vi "Calculator Brainstorming V4.vi"() -> ()   [LabVIEW 2017]
doc: "This is a calculator designed for physics students. It features 7 commonly used physics constants, and the 4 usual operators."
panel:
  in  "=":bool
  in  "÷":bool
  in  "x":bool
  in  "-":bool
  in  "+":bool
  in  "0 8":bool
  in  "Pi":bool
  in  "0 7":bool
  in  "mp":bool
  in  "me":bool
  in  "G":bool
  in  "C":bool
  in  ".":bool
  in  "9":bool
  in  "8":bool
  in  "7":bool
  in  "0":bool
  in  "6":bool
  in  "?":bool
  in  "?":bool
  in  "1":bool
  in  "5":bool
  in  "4":bool
  in  "3":bool
  in  "2":bool
  out "Display":dbl
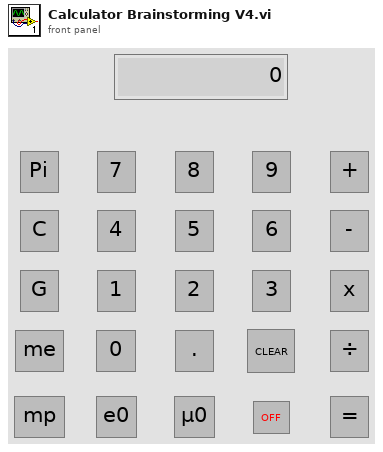
[diagram p1: front panel]
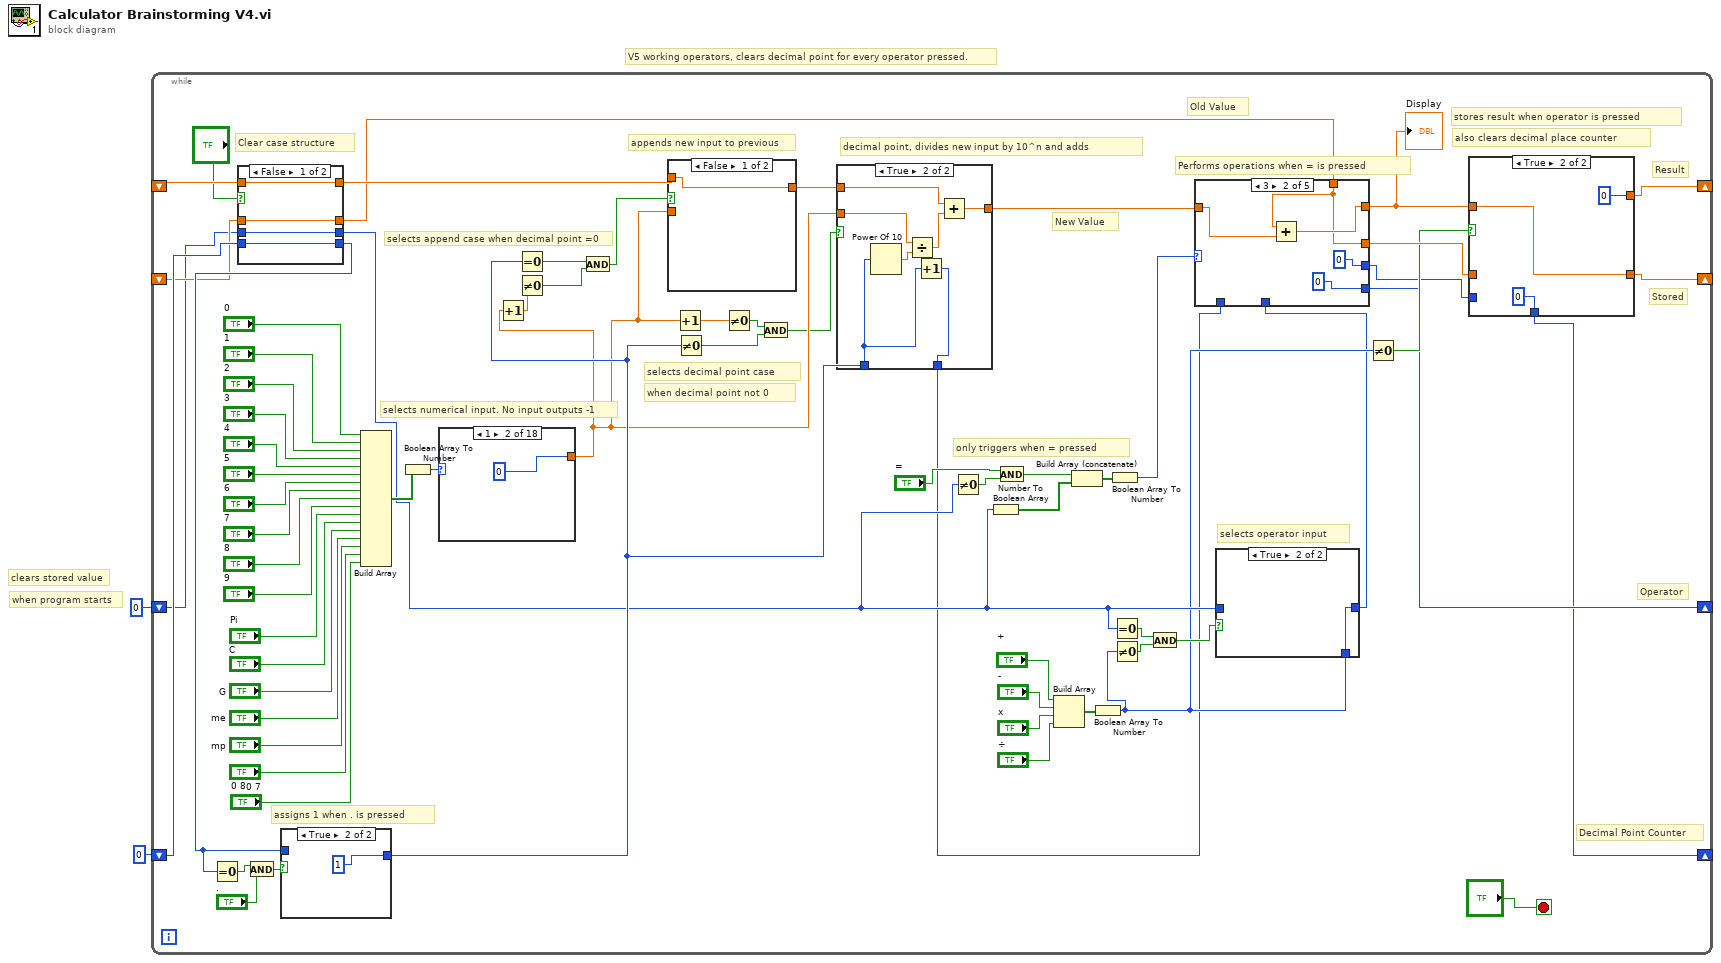
[diagram p0: block diagram]
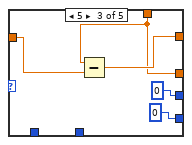
[diagram p4: hidden frame]
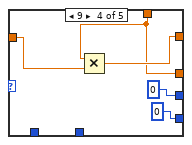
[diagram p5: hidden frame]
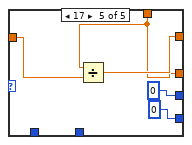
[diagram p6: hidden frame]
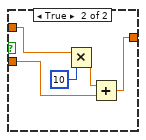
[diagram p8: hidden frame]
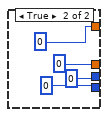
[diagram p11: hidden frame]
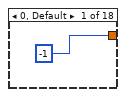
[diagram p12: hidden frame]
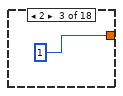
[diagram p13: hidden frame]
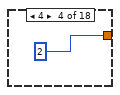
[diagram p14: hidden frame]
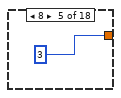
[diagram p15: hidden frame]
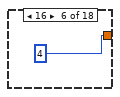
[diagram p16: hidden frame]
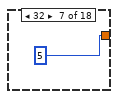
[diagram p17: hidden frame]
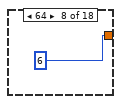
[diagram p18: hidden frame]
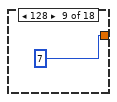
[diagram p19: hidden frame]
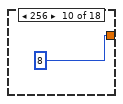
[diagram p20: hidden frame]
diagram:
  # "when program starts"
  # "clears stored value"
  # "V5 working operators, clears decimal point for every operator pressed."
  n1 = while {
    shift-right: [w16] -> _
    shift-left: _ -> [w69]
    shift-right: [w4] -> _
    shift-left: 0 -> [w52]
    shift-right: [w17] -> _
    shift-left: _ -> [w34]
    shift-right: [w7] -> _
    shift-left: 0 -> [w32]
    stop <- "?" stop-if-true
    # "Clear case structure"
    # "when decimal point not 0"
    # "selects decimal point case"
    # "selects append case when decimal point =0"
    # "also clears decimal place counter"
    # "stores result when operator is pressed"
    # "Performs operations when = is pressed"
    # "assigns 1 when . is pressed"
    # "only triggers when = pressed"
    # "selects operator input"
    # "decimal point, divides new input by 10^n and adds"
    # "New Value"
    # "Old Value"
    # "Operator"
    # "Stored"
    # "Decimal Point Counter"
    # "appends new input to previous"
    # "selects numerical input. No input outputs -1"
    # "Result"
    n2 = case shown="False" "?" {
      tunnel: [w124 0] -> w33
      tunnel: w69 -> [w124 _]
      tunnel: [w123 0] -> w53
      tunnel: w52 -> [w123 _]
      tunnel: [w122 0] -> w27
      tunnel: w34 -> [w122 _]
      tunnel: [w121 0] -> w12
      tunnel: w32 -> [w121 _]
      frame False {
      }
      frame True {
      }
    }
    n3 = Equal To 0?(x=w53) -> (x = 0?=w55:bool)
    n4 = And(x=w55, y=".") -> (x .and. y?=w56:bool)
    n5 = case shown="True" w56 {
      tunnel: w53 -> [w119 _]
      tunnel: [w119 1] -> w47
      frame False {
      }
      frame True {
      }
    }
    n6 = Build Array("0", "1", "2", "3", "4", "5", "6", "7", "8", "9", "Pi", "C", "G", "me", "mp", "0 7", "0 8") -> (w67:bool[])
    n7 = Boolean Array To Number(Boolean array=w67) -> (number=w71:u32)
    n8 = case shown="1" w71 {
      tunnel: [-1 0 1 2 3 4 5 6 7 8 9 3.141592653589793 w142 w144 9.10938356e-31 1.6726219e-27 8.85418782e-12 1.25663706e-06] -> w46
      frame 0, Default {
      }
      frame 1 {
      }
      frame 2 {
      }
      frame 4 {
      }
      frame 8 {
      }
      frame 16 {
      }
      frame 32 {
      }
      frame 64 {
      }
      frame 128 {
      }
      frame 256 {
      }
      frame 512 {
      }
      frame 1024 {
      }
      frame 2048 {
        # "cast to remove units"
        n9 = Cast Unit Bases(0:ext[unit] 299792458.0) -> (2:w142:ext)  [unwired: 1 in]
      }
      frame 4096 {
        n10 = Cast Unit Bases(0:ext[unit] 6.67408e-11) -> (2:w144:ext)  [unwired: 1 in]
      }
      frame 8192 {
      }
      frame 16384 {
      }
      frame 32768 {
      }
      frame 65536 {
      }
    }
    n11 = Increment(x=w46) -> (x+1=w49:ext)
    n12 = Equal To 0?(x=w47) -> (x = 0?=w48:bool)
    n13 = Not Equal To 0?(x=w49) -> (x != 0?=w50:bool)
    n14 = And(x=w48, y=w50) -> (x .and. y?=w3:bool)
    n15 = case shown="False" w3 {
      tunnel: w33 -> [w104 w107]
      tunnel: [w104 w106] -> w51
      tunnel: w46 -> [_ w105]
      frame False {
      }
      frame True {
        n16 = Multiply(x=w107, y=10) -> (x*y=w109:ext)
        n17 = Add(x=w109, y=w105) -> (x+y=w106:ext)
      }
    }
    n18 = Increment(x=w46) -> (x+1=w42:ext)
    n19 = Not Equal To 0?(x=w47) -> (x != 0?=w44:bool)
    n20 = Not Equal To 0?(x=w42) -> (x != 0?=w45:bool)
    n21 = And(x=w45, y=w44) -> (x .and. y?=w43:bool)
    n22 = case shown="True" w43 {
      tunnel: w51 -> [w111 w116]
      tunnel: [w111 w115] -> w23
      tunnel: w47 -> [w110 w113]
      tunnel: w46 -> [_ w114]
      tunnel: [w110 w112] -> w6
      frame False {
      }
      frame True {
        n23 = Power Of 10(x=w113) -> (10^x=w118:dbl)
        n24 = Divide(x=w114, y=w118) -> (x/y=w117:ext)
        n25 = Increment(x=w113) -> (x+1=w112:i32)
        n26 = Add(x=w116, y=w117) -> (x+y=w115:ext)
      }
    }
    n27 = Not Equal To 0?(x=w12) -> (x != 0?=w25:bool)
    n28 = Number To Boolean Array(number=w12) -> (Boolean array=w22:bool[])
    n29 = And(x="=", y=w25) -> (x .and. y?=w21:bool)
    n30 = Build Array("+", "-", "x", "÷") -> (w26:bool[])
    n31 = Build Array (concatenate)(w21, w22) -> (w20:bool[])
    n32 = Boolean Array To Number(Boolean array=w26) -> (number=w10:u32)
    n33 = Boolean Array To Number(Boolean array=w20) -> (number=w19:u32)
    n34 = Equal To 0?(x=w12) -> (x = 0?=w14:bool)
    n35 = Not Equal To 0?(x=w10) -> (x != 0?=w11:bool)
    n36 = And(x=w14, y=w11) -> (x .and. y?=w13:bool)
    n37 = case shown="True" w13 {
      tunnel: w12 -> [w102 _]
      tunnel: [w102 w103] -> w8
      tunnel: w10 -> [_ w103]
      frame False {
      }
      frame True {
      }
    }
    n38 = case shown="3" w19 {
      tunnel: [w80 w86 w91 w96 w101] -> w18
      tunnel: w27 -> [w81 w84 w89 w94 w99]
      tunnel: [w81 w84 w89 w94 w99] -> w15
      tunnel: w23 -> [w80 w85 w90 w95 w100]
      tunnel: w8 -> [w79 _ _ _ _]
      tunnel: [w79 0 0 0 0] -> w7
      tunnel: w6 -> [w78 _ _ _ _]
      tunnel: [w78 0 0 0 0] -> w5
      frame 0, Default {
      }
      frame 3 {
        n39 = Add(x=w84, y=w85) -> (x+y=w86:ext)
      }
      frame 5 {
        n40 = Subtract(x=w89, y=w90) -> (x-y=w91:ext)
      }
      frame 9 {
        n41 = Multiply(x=w94, y=w95) -> (x*y=w96:ext)
      }
      frame 17 {
        n42 = Divide(x=w99, y=w100) -> (x/y=w101:ext)
      }
    }
    "Display" <- w18
    n43 = Not Equal To 0?(x=w10) -> (x != 0?=w9:bool)
    n44 = case shown="True" w9 {
      tunnel: w18 -> [w74 w77]
      tunnel: [w73 w77] -> w17
      tunnel: [w74 0] -> w16
      tunnel: w15 -> [w73 _]
      tunnel: w5 -> [w72 _]
      tunnel: [w72 0] -> w4
      frame False {
      }
      frame True {
      }
    }
  }
